vi "Load Flattened 32bit float Image from Tiff.vi"(0 "path to TIFF file":path=path "/HD1/Users/herbertlooser/Desktop/LadungssprŸher.tif", 1 "error in (no error)":errorcluster, 2 "Image Index":i32) -> (5 "Gray16/32":sgl[][](array[numeric]), 7 "error out":errorcluster)   [LabVIEW 2013, in "Tiff reader.lvlib"]
doc: "This .vi is taken from an online tiff reader. It is able to read 32-bit floating point .tiff images."
uses:
  Tiff reader.lvlib
  Bytes to word.vi
  Bytes to long word.vi
panel:
  out "Intensity Graph":sgl[][](graph)
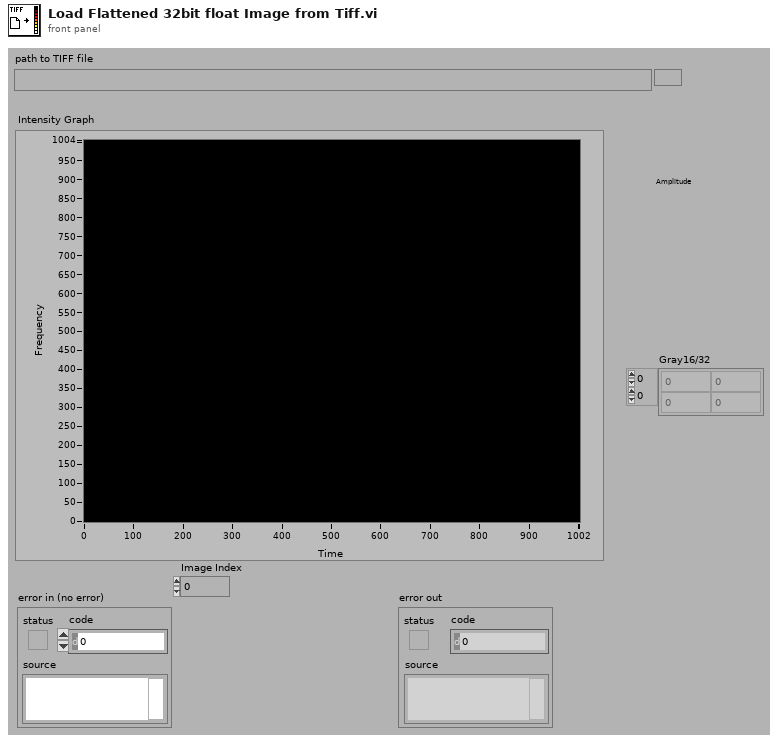
[diagram p1: front panel]
types:
  T1 = enum16{"open", "open or create", "create or replace", "create"}
  T2 = typedef "Tiff reader.lvlib/IFD Entry.ctl" = cluster{"Tag":u16, "Type":T3, "Count":u32, "Val/Offs":u32, "Is Pointer?":bool, "Byte stream index":i32}
  T3 = typedef "Tiff reader.lvlib/FieldTypes.ctl" = enum16{"NULL", "U8", "ASCII7", "U16", "U32", "RATIONAL", "SByte(I8)", "Undef(8Bit)", "I16", "I32", "SRat(4B:4B)", "SGL(4Byte)", "DBL(8Byte)"}
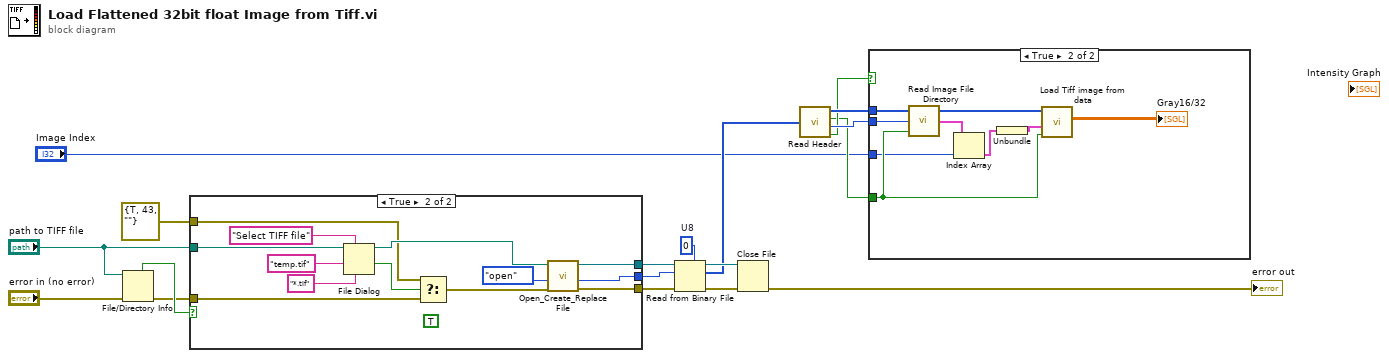
[diagram p0: block diagram]
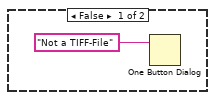
[diagram p2: hidden frame]
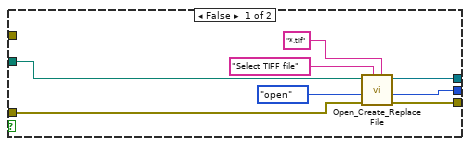
[diagram p3: hidden frame]
diagram:
  w3 = u8 0  # U8
  n1 = File/Directory Info(path="path to TIFF file", error in="error in (no error)") -> (directory=w13:bool, error out=w4:errorcluster)  [unwired: 5 out]
  n2 = case shown="True" w13 {
    tunnel: [w23 w32] -> w18
    tunnel: [w22 w34] -> w17
    tunnel: [w21 w33] -> w14
    tunnel: w4 -> [w20 w30]
    tunnel: "path to TIFF file" -> [w19 w27]
    tunnel: errorcluster {"status"=TRUE, "code"=43, "source"=""} ("error in (no error)") -> [_ w28]
    frame False {
      n3 = call <vilib>:"Open_Create_Replace File.vi"("pattern"="*.tif", "prompt"="Select TIFF file", "error in (no error)"=w20, "function (open:0)"=T1."open", "file path"=w19) -> ("error out"=w21:errorcluster, "file size (bytes)"=w23:i32, "refnum"=w22:refnum<file>)  [unwired: 2 in, 2 out]
    }
    frame True {
      (unwired) TRUE ("advisory dialog? (display:T)")
      n4 = File Dialog(6:"*.tif" ("pattern"), 7:"Select TIFF file" ("prompt"), 9:"temp.tif" ("default name"), 11:w27) -> (1:w31:bool, 3:w36:path)  [unwired: 1 in, 4 out]
      n5 = Select(t=w28, s=w31, f=w30) -> (s? t:f=w29:errorcluster)
      n6 = call <vilib>:"Open_Create_Replace File.vi"("error in (no error)"=w29, "function (open:0)"=T1."open", "file path"=w36) -> ("error out"=w33:errorcluster, "file size (bytes)"=w32:i32, "refnum"=w34:refnum<file>)  [unwired: 3 in, 3 out]
    }
  }
  n7 = Read from Binary File(5:w3, 8:w14, 10:w18, 11:w17) -> (0:w15:errorcluster, 2:w2:u8[], 3:w16:refnum<file>)  [unwired: 3 out]
  n8 = Close File(refnum=w16, error in=w15) -> (error out=→"error out":errorcluster)  [unwired: 1 out]
  n9 = call "Read Header.vi"("TIFF Data in"=w2) -> ("TIFF Data out"=w10:u8[], "Litt/BigEnd"=w7:bool, "ImFileDirectOffs"=w9:u32, "IsTIFF?"=w8:bool)
  n10 = case shown="True" w8 {
    tunnel: w10 -> [_ w49]
    tunnel: w9 -> [_ w48]
    tunnel: w7 -> [_ w46]
    tunnel: "Image Index" -> [_ w41]
    frame False {
      n11 = One Button Dialog(message="Not a TIFF-File") -> ()  [unwired: 2 out]
    }
    frame True {
      n12 = call "Read Image File Directory.vi"("Litt/BigEnd"=w46, "Im_File_Dir Offs"=w48, "Image Data in"=w49) -> ("Directories"=w45:cluster{"Tags":T2[]}[], "Image Data out"=w47:u8[])  [unwired: 1 out]
      n13 = Index Array(array=w45, index=w41) -> (element=w43:cluster{"Tags":T2[]})
      n14 = Unbundle(w43) -> ("Tags"=w42:T2[])
      n15 = call "Load Tiff image from data.vi"("Litt/BigEnd"=w46, "DirEntries"=w42, "Image Data in"=w47) -> ("Gray16/32"=→"Gray16/32":sgl[][])  [unwired: 8 out]
    }
  }
